vi "VIrefParse.vi"(3 "Var Number":dbl, 4 "VIA":string, 5 "Params":T1, 6 "String in":string) -> (0 "Var Number 2":dbl, 1 "defaults":string, 2 "String out":string)   [LabVIEW 2012]
panel:
  out "Array":string[](array[string])
  out "Array 2":T2(array[cluster])
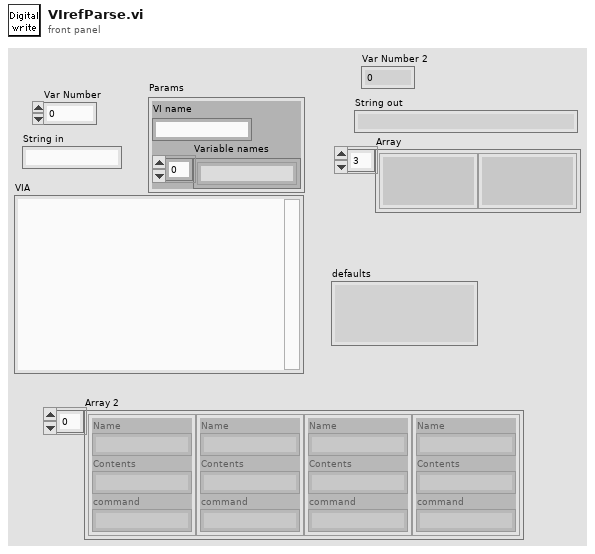
[diagram p1: front panel]
types:
  T1 = cluster{"VI name":string, "Variable names":string[]}
  T2 = cluster{"Name":string, "Contents":string, "command":string}[]
  T3 = cluster{"trimmed string":string, "Contents":string, "command":string}
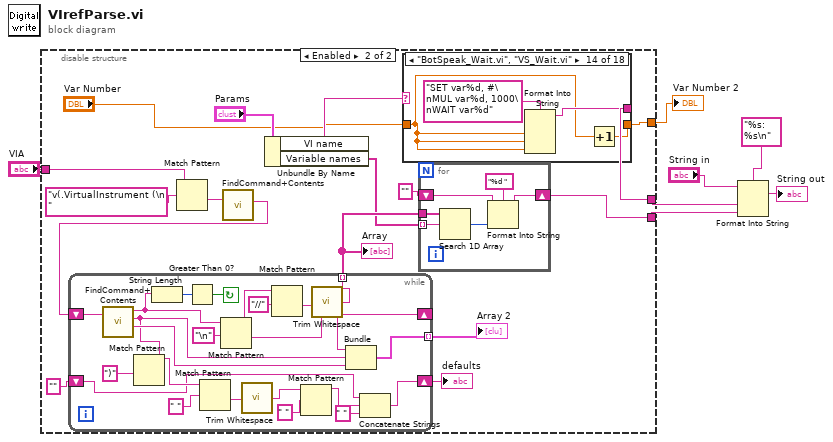
[diagram p0: block diagram]
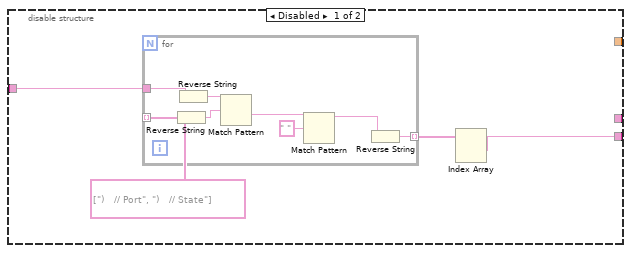
[diagram p2: hidden frame]
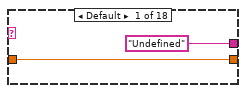
[diagram p3: hidden frame]
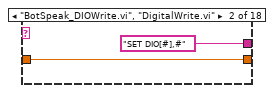
[diagram p4: hidden frame]
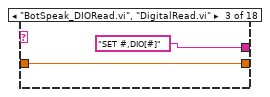
[diagram p5: hidden frame]
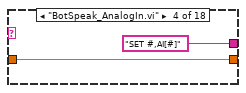
[diagram p6: hidden frame]
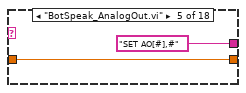
[diagram p7: hidden frame]
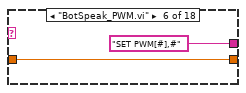
[diagram p8: hidden frame]
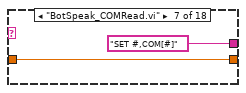
[diagram p9: hidden frame]
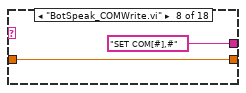
[diagram p10: hidden frame]
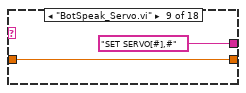
[diagram p11: hidden frame]
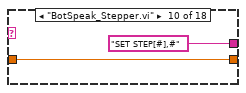
[diagram p12: hidden frame]
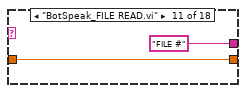
[diagram p13: hidden frame]
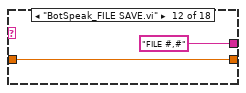
[diagram p14: hidden frame]
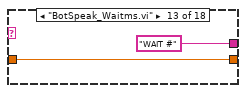
[diagram p15: hidden frame]
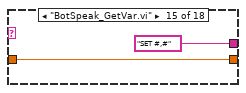
[diagram p16: hidden frame]
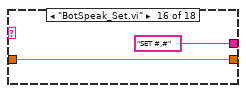
[diagram p17: hidden frame]
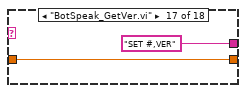
[diagram p18: hidden frame]
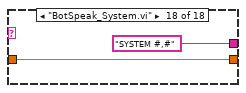
[diagram p19: hidden frame]
diagram:
  n1 = disable-structure shown="Enabled" {
    disable-tunnel: "VIA" -> [w12 w35]
    disable-tunnel: [w9 w28] -> w3
    disable-tunnel: [_ w26] -> w2
    disable-tunnel: [_ w21] -> w1
    frame Disabled {
      n2 = for {
        tunnel: w12 -> [w20]
        tunnel: [w15] -> w10 mode=indexing
        tunnel: string[] [")   // Port", ")   // State"] -> [w13] mode=indexing
        n3 = Reverse String(1:w13) -> (0:w18:string)
        n4 = Reverse String(1:w20) -> (0:w19:string)
        n5 = Match Pattern(string=w19, regular expression=w18) -> (after substring=w16:string)  [unwired: 1 in, 3 out]
        n6 = Match Pattern(string=w16, regular expression=" ") -> (before substring=w14:string)  [unwired: 1 in, 3 out]
        n7 = Reverse String(1:w14) -> (0:w15:string)
      }
      n8 = Index Array(array=w10) -> (element #1=w9:string, element #2=w8:string)  [unwired: 2 in]
    }
    frame Enabled {
      n9 = Match Pattern(string=w35, regular expression="v(.VirtualInstrument (\n   ") -> (after substring=w34:string)  [unwired: 1 in, 3 out]
      n10 = call <userlib>:"FindCommand+Contents.vi"("Via file in"=w34) -> ("Contents"=w33:string)  [unwired: 1 in, 3 out]
      n11 = while {
        shift-right: [w97] -> _
        shift-left: w33 -> [w103]
        tunnel: [w99] -> w25 mode=indexing
        tunnel: [w92] -> w32 mode=indexing
        shift-right: [w82] -> w23
        shift-left: "" -> [w84]
        stop <- w101 continue-if-true
        n12 = call <userlib>:"FindCommand+Contents.vi"("Via file in"=w103) -> ("left"=w96:string, "Contents"=w85:string, "command"=w100:string)  [unwired: 1 in, 1 out]
        n13 = Match Pattern(string=w85, regular expression=")") -> (before substring=w90:string)  [unwired: 1 in, 3 out]
        n14 = String Length(string=w96) -> (length=w102:i32)
        n15 = Greater Than 0?(x=w102) -> (x > 0?=w101:bool)
        n16 = Match Pattern(string=w90, regular expression=" ") -> (after substring=w88:string)  [unwired: 1 in, 3 out]
        n17 = Match Pattern(string=w96, regular expression="\n") -> (before substring=w95:string, after substring=w97:string)  [unwired: 1 in, 2 out]
        n18 = call <vilib>:"Trim Whitespace.vi"("string"=w88) -> ("trimmed string"=w87:string)  [unwired: 1 in]
        n19 = Match Pattern(string=w95, regular expression="//") -> (after substring=w94:string)  [unwired: 1 in, 3 out]
        n20 = Match Pattern(string=w87, regular expression=" ") -> (before substring=w83:string)  [unwired: 1 in, 3 out]
        n21 = call <vilib>:"Trim Whitespace.vi"("string"=w94) -> ("trimmed string"=w92:string)  [unwired: 1 in]
        n22 = Bundle("trimmed string"=w92, "Contents"=w85, "command"=w100) -> (w99:T3)  [unwired: 1 in]
        n23 = Concatenate Strings(w84, w83, " " ("string")) -> (w82:string)
      }
      "Array 2" <- w25
      "Array" <- w32
      "defaults" <- w23
      n24 = Unbundle By Name("Params") -> ("VI name"=w27:string, "Variable names"=w30:string[])
      n25 = case shown="\"BotSpeak_Wait.vi\", \"VS_Wait.vi\"" w27 {
        tunnel: ["Undefined" ("format string") "SET DIO[#],#" ("format string") "SET #,DIO[#]" ("format string") "SET #,AI[#]" ("format string") "SET AO[#],#" ("format string") "SET PWM[#],#" ("format string") "SET #,COM[#]" ("format string") "SET COM[#],#" ("format string") "SET SERVO[#],#" ("format string") "SET STEP[#],#" ("format string") "FILE #" ("format string") "FILE #,#" ("format string") "WAIT #" ("format string") w64 "SET #,#" ("format string") "SET #,#" ("format string") "SET #,VER" ("format string") "SYSTEM #,#" ("format string")] -> w26
        tunnel: "Var Number" -> [w37 w39 w41 w43 w45 w47 w49 w51 w53 w55 w57 w59 w61 w63 w67 w69 w71 w73]
        tunnel: [w37 w39 w41 w43 w45 w47 w49 w51 w53 w55 w57 w59 w61 w66 w67 w69 w71 w73] -> w21
        frame Default {
        }
        frame "BotSpeak_DIOWrite.vi", "DigitalWrite.vi" {
        }
        frame "BotSpeak_DIORead.vi", "DigitalRead.vi" {
        }
        frame "BotSpeak_AnalogIn.vi" {
        }
        frame "BotSpeak_AnalogOut.vi" {
        }
        frame "BotSpeak_PWM.vi" {
        }
        frame "BotSpeak_COMRead.vi" {
        }
        frame "BotSpeak_COMWrite.vi" {
        }
        frame "BotSpeak_Servo.vi" {
        }
        frame "BotSpeak_Stepper.vi" {
        }
        frame "BotSpeak_FILE READ.vi" {
        }
        frame "BotSpeak_FILE SAVE.vi" {
        }
        frame "BotSpeak_Waitms.vi" {
        }
        frame "BotSpeak_Wait.vi", "VS_Wait.vi" {
          n26 = Format Into String(format string="SET var%d, #\nMUL var%d, 1000\nWAIT var%d", w63, w63, w63) -> (resulting string=w64:string)  [unwired: 2 in, 1 out]
          n27 = Increment(x=w63) -> (x+1=w66:dbl)
        }
        frame "BotSpeak_GetVar.vi" {
        }
        frame "BotSpeak_Set.vi" {
        }
        frame "BotSpeak_GetVer.vi" {
        }
        frame "BotSpeak_System.vi" {
        }
      }
      n28 = for {
        tunnel: w30 -> [w80] mode=indexing
        tunnel: w32 -> [w78]
        shift-right: [w76] -> w28
        shift-left: "" -> [w75]
        n29 = Search 1D Array(1D array=w78, element=w80) -> (index of element=w79:i32)  [unwired: 1 in]
        n30 = Format Into String(format string="%d ", initial string=w75, w79) -> (resulting string=w76:string)  [unwired: 1 in, 1 out]
      }
    }
  }
  "Var Number 2" <- w1
  n31 = Format Into String(format string="%s: %s\n" ("regular expression"), initial string="String in", w2, w3) -> (resulting string=→"String out":string)  [unwired: 1 in, 1 out]
